vi "Produce error Cluster.vi"() -> (0 "Error Bar Cluster":T1[](array[typedef]))   [LabVIEW 2018]
uses:
  Error_bars.ctl
  Results_plotter_Global.vi
  Data plotting/subVIs/RFP_Table_Global.vi
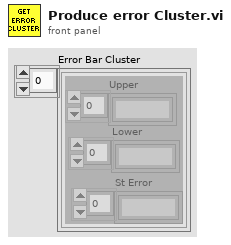
[diagram p1: front panel]
types:
  T1 = typedef "Error_bars.ctl" = cluster{"Upper":string[], "Lower":string[], "St Error":string[]}
  T2 = typedef "RFP_Plot_Metadata.ctl" = cluster{"Row Number":i32[], "Error Bars":T3, "X Label":string, "Y Label":string}
  T3 = typedef "Error_bars_index.ctl" = cluster{"Upper":i32, "Lower":i32, "St Error":i32}
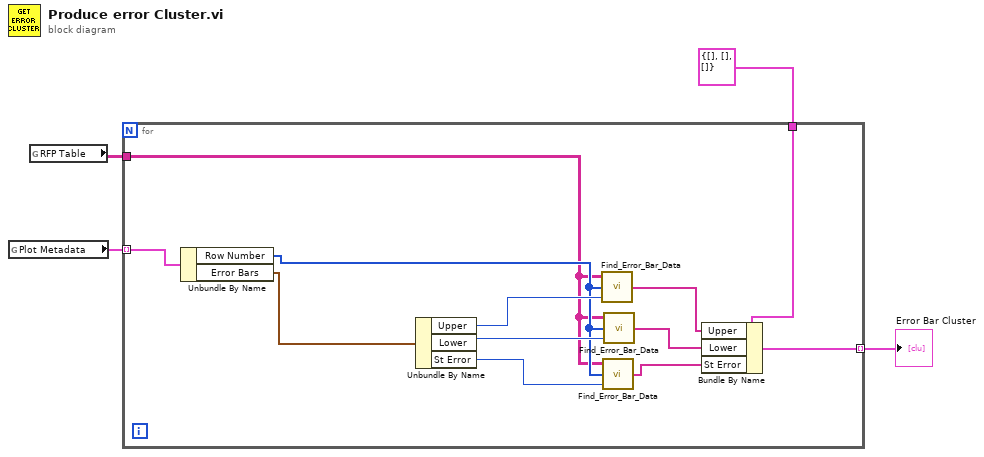
[diagram p0: block diagram]
diagram:
  n1 = global read "Results_plotter_Global.vi" "Plot Metadata"() -> (w4:T2[])
  n2 = global read "RFP_Table_Global.vi" "RFP Table"() -> (w1:string[][])
  n3 = for {
    tunnel: w1 -> [w7]
    tunnel: w4 -> [w16] mode=indexing
    tunnel: T1 {"Upper"=[], "Lower"=[], "St Error"=[]} ("Error_bars") -> [w6]
    tunnel: [w5] -> w2 mode=indexing
    n4 = Unbundle By Name(w16) -> ("Row Number"=w8:i32[], "Error Bars"=w9:T3)
    n5 = Unbundle By Name(w9) -> ("Upper"=w11:i32, "Lower"=w12:i32, "St Error"=w13:i32)
    n6 = call "Find_Error_Bar_Data.vi"("Ch Index"=w11, "Row Numbers"=w8, "Channel Values"=w7) -> ("Error bar values"=w10:string[])
    n7 = call "Find_Error_Bar_Data.vi"("Ch Index"=w13, "Row Numbers"=w8, "Channel Values"=w7) -> ("Error bar values"=w14:string[])
    n8 = call "Find_Error_Bar_Data.vi"("Ch Index"=w12, "Row Numbers"=w8, "Channel Values"=w7) -> ("Error bar values"=w15:string[])
    n9 = Bundle By Name(cluster=w6, "Upper"=w10, "Lower"=w15, "St Error"=w14) -> (w5:T1)
  }
  "Error Bar Cluster" <- w2
